vi "Main_flow_full_mqtt.vi"() -> ()   [LabVIEW 2022 SP3]
uses:
  D:/UOM/EE2044 - Electrical Measurements and Instrumentation/Project/Measurment Project/Quaxo_MQTT_LabVIEW-master/Controls/QoS.ctl
  D:/UOM/EE2044 - Electrical Measurements and Instrumentation/Project/Measurment Project/Quaxo_MQTT_LabVIEW-master/Controls/Retain_Flag.ctl
  D:/UOM/EE2044 - Electrical Measurements and Instrumentation/Project/Measurment Project/Quaxo_MQTT_LabVIEW-master/Controls/DUP_Flag.ctl
  D:/UOM/EE2044 - Electrical Measurements and Instrumentation/Project/Measurment Project/Quaxo_MQTT_LabVIEW-master/Controls/Connection_Return_Codes.ctl
  D:/UOM/EE2044 - Electrical Measurements and Instrumentation/Project/Measurment Project/Quaxo_MQTT_LabVIEW-master/Controls/Connect_Flags.ctl
  D:/UOM/EE2044 - Electrical Measurements and Instrumentation/Project/Measurment Project/Quaxo_MQTT_LabVIEW-master/Controls/User_Info.ctl
  <vilib>/DAQmx/write.llb/DAQmx Write (Digital Bool 1Line 1Point).vi
  <vilib>/DAQmx/read.llb/DAQmx Read (Digital Bool 1Line 1Point).vi
  <vilib>/DAQmx/read.llb/DAQmx Read (Analog 1D DBL NChan 1Samp).vi
  <vilib>/DAQmx/create/channels.llb/DAQmx Create Channel (AI-Voltage-Basic).vi
  <vilib>/DAQmx/create/channels.llb/DAQmx Create Channel (DO-Digital Output).vi
  <vilib>/DAQmx/create/channels.llb/DAQmx Create Channel (DI-Digital Input).vi
  <vilib>/DAQmx/miscellaneous.llb/DAQmx Fill In Error Info.vi
  D:/UOM/EE2044 - Electrical Measurements and Instrumentation/Project/Measurment Project/Quaxo_MQTT_LabVIEW-master/MQTT_Functions.lvlib
panel:
  out "Connection Status":T1=enum."Connection refused: not authorized"
  in  "Stop Publishing":bool
  out "Message published":string
  out "Acknowledged":bool
  out "Message ID (acknowledged)":u16=10
  in  "Message ID":u16=20
  in  "MQTT Broker":cluster{"address (IP)":string, "port":u16}={"address (IP)"="broker.mqttdashboard.com", "port"=1883}
  in  "Message to be published":string="Quaxo says it's "
  out "error out":errorcluster
  in  "Client ID":string="NodeE-12345"
  in  "error in (no error)":errorcluster
  in  "Topic":string="testtopic/Node12345"
  in  "Publish Meta":cluster{"QoS":T2, "Retain":T3, "DUP":T4}
  out "main loop executed":dbl
  out "Servo Angle":dbl(slide) scale=0.0..150.0
  in  "stop (F)":bool
  out "Square":dynamicdata(graph)
  in  "Frequency":dbl=50.0
  in  "Offset":dbl=2.5
  in  "Amplitude":dbl=2.5
  out "LDR Value":dbl
  in  "Relay 2":tag
  in  "Relay 1":tag
  out "Numeric 2":dbl
  out "Numeric":dbl
  in  "UP DOWN 2":tag
  in  "UP DOWN 1":tag
  in  "Buzzer":tag
  out "Counter":dbl
  out "OUT COUNT":dbl
  out "IN COUNT":dbl
  in  "Door IR 1 & 2 & LDR":tag
  in  "Trigger Period(sec)":dbl
  out "Current Time":dbl
  in  "Mode":dbl
  in  "stop":bool
  # "Dev1/ai4:6"
  # "Dev1/port0/line2"
  # "Dev1/port0/line0"
  # "Dev1/port0/line1"
  # "Dev1/port0/line3"
  # "Dev1/port0/line3"
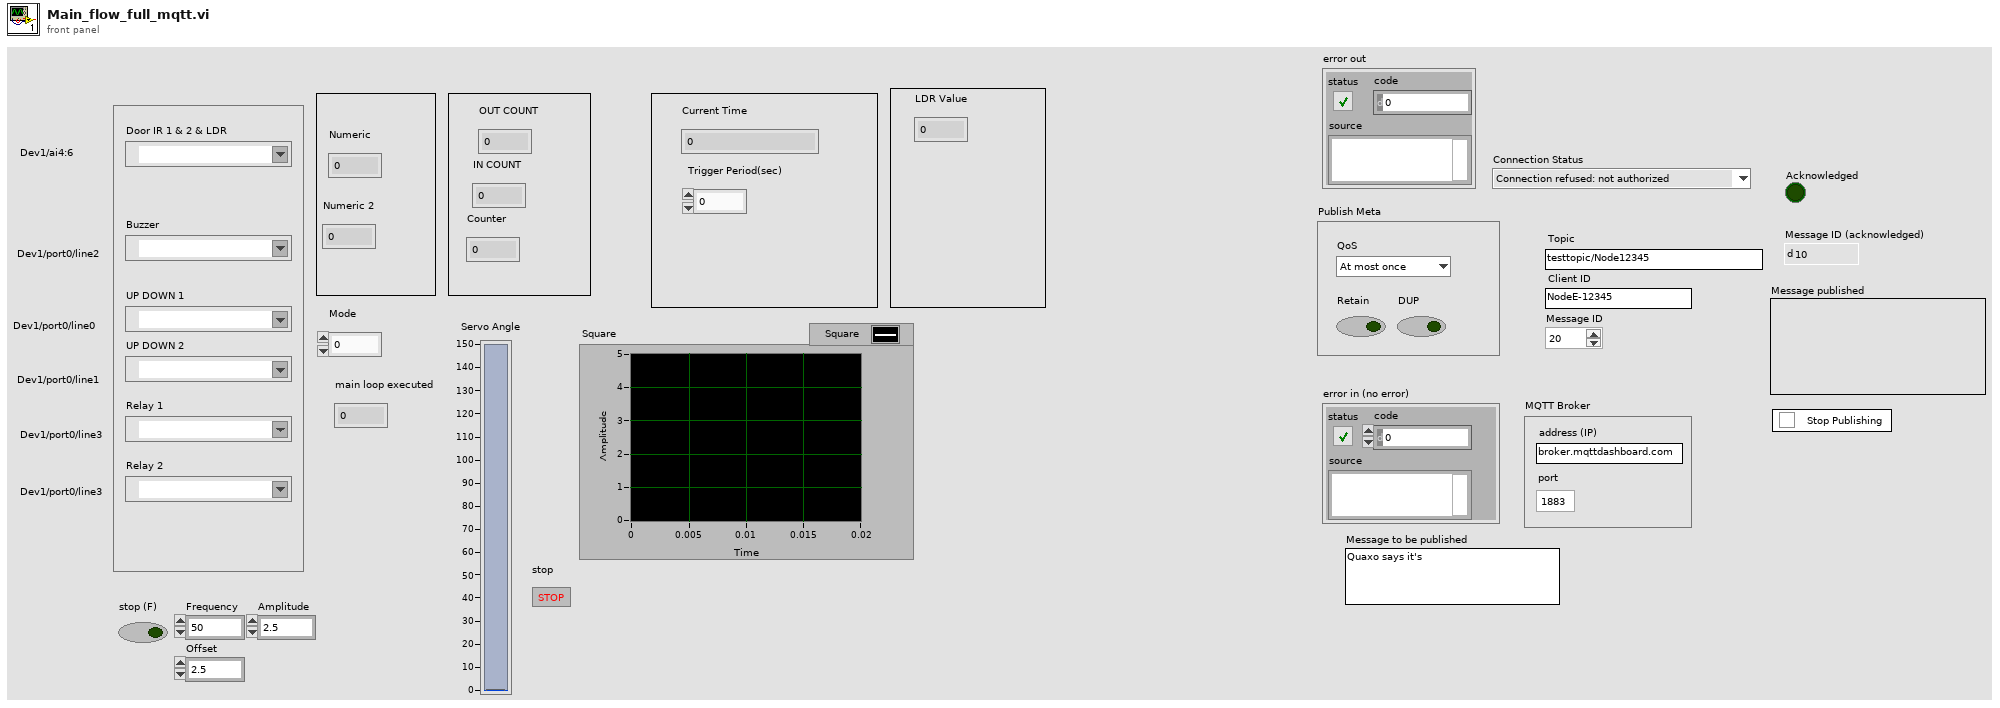
[diagram p1: front panel]
types:
  T1 = typedef "MQTT_Functions.lvlib/Connection_Return_Codes.ctl" = enum16{"Connection accepted", "Connection refused: unacceptable protocol version", "Connection refused: identifier rejected", "Connection refused: Server unavailable", "Connection refused: bad user name or password", "Connection refused: not authorized"}
  T2 = typedef "MQTT_Functions.lvlib/QoS.ctl" = enum8{"At most once", "At least once", "Exactly once", "Reserved"}
  T3 = typedef "MQTT_Functions.lvlib/Retain_Flag.ctl" = bool
  T4 = typedef "MQTT_Functions.lvlib/DUP_Flag.ctl" = bool
  T5 = typedef "MQTT_Functions.lvlib/User_Info.ctl" = cluster{"User Name":string, "Password":string}
  T6 = typedef "MQTT_Functions.lvlib/Connect_Flags.ctl" = cluster{"user name":bool, "password":bool, "will retain":bool, "will flag":bool, "clean session":bool, "reserved":bool, "will QoS":T2}
  T7 = cluster{"QoS":T2, "DUP":T4, "Retain":T3, "Keep Alive (sec)":u16}
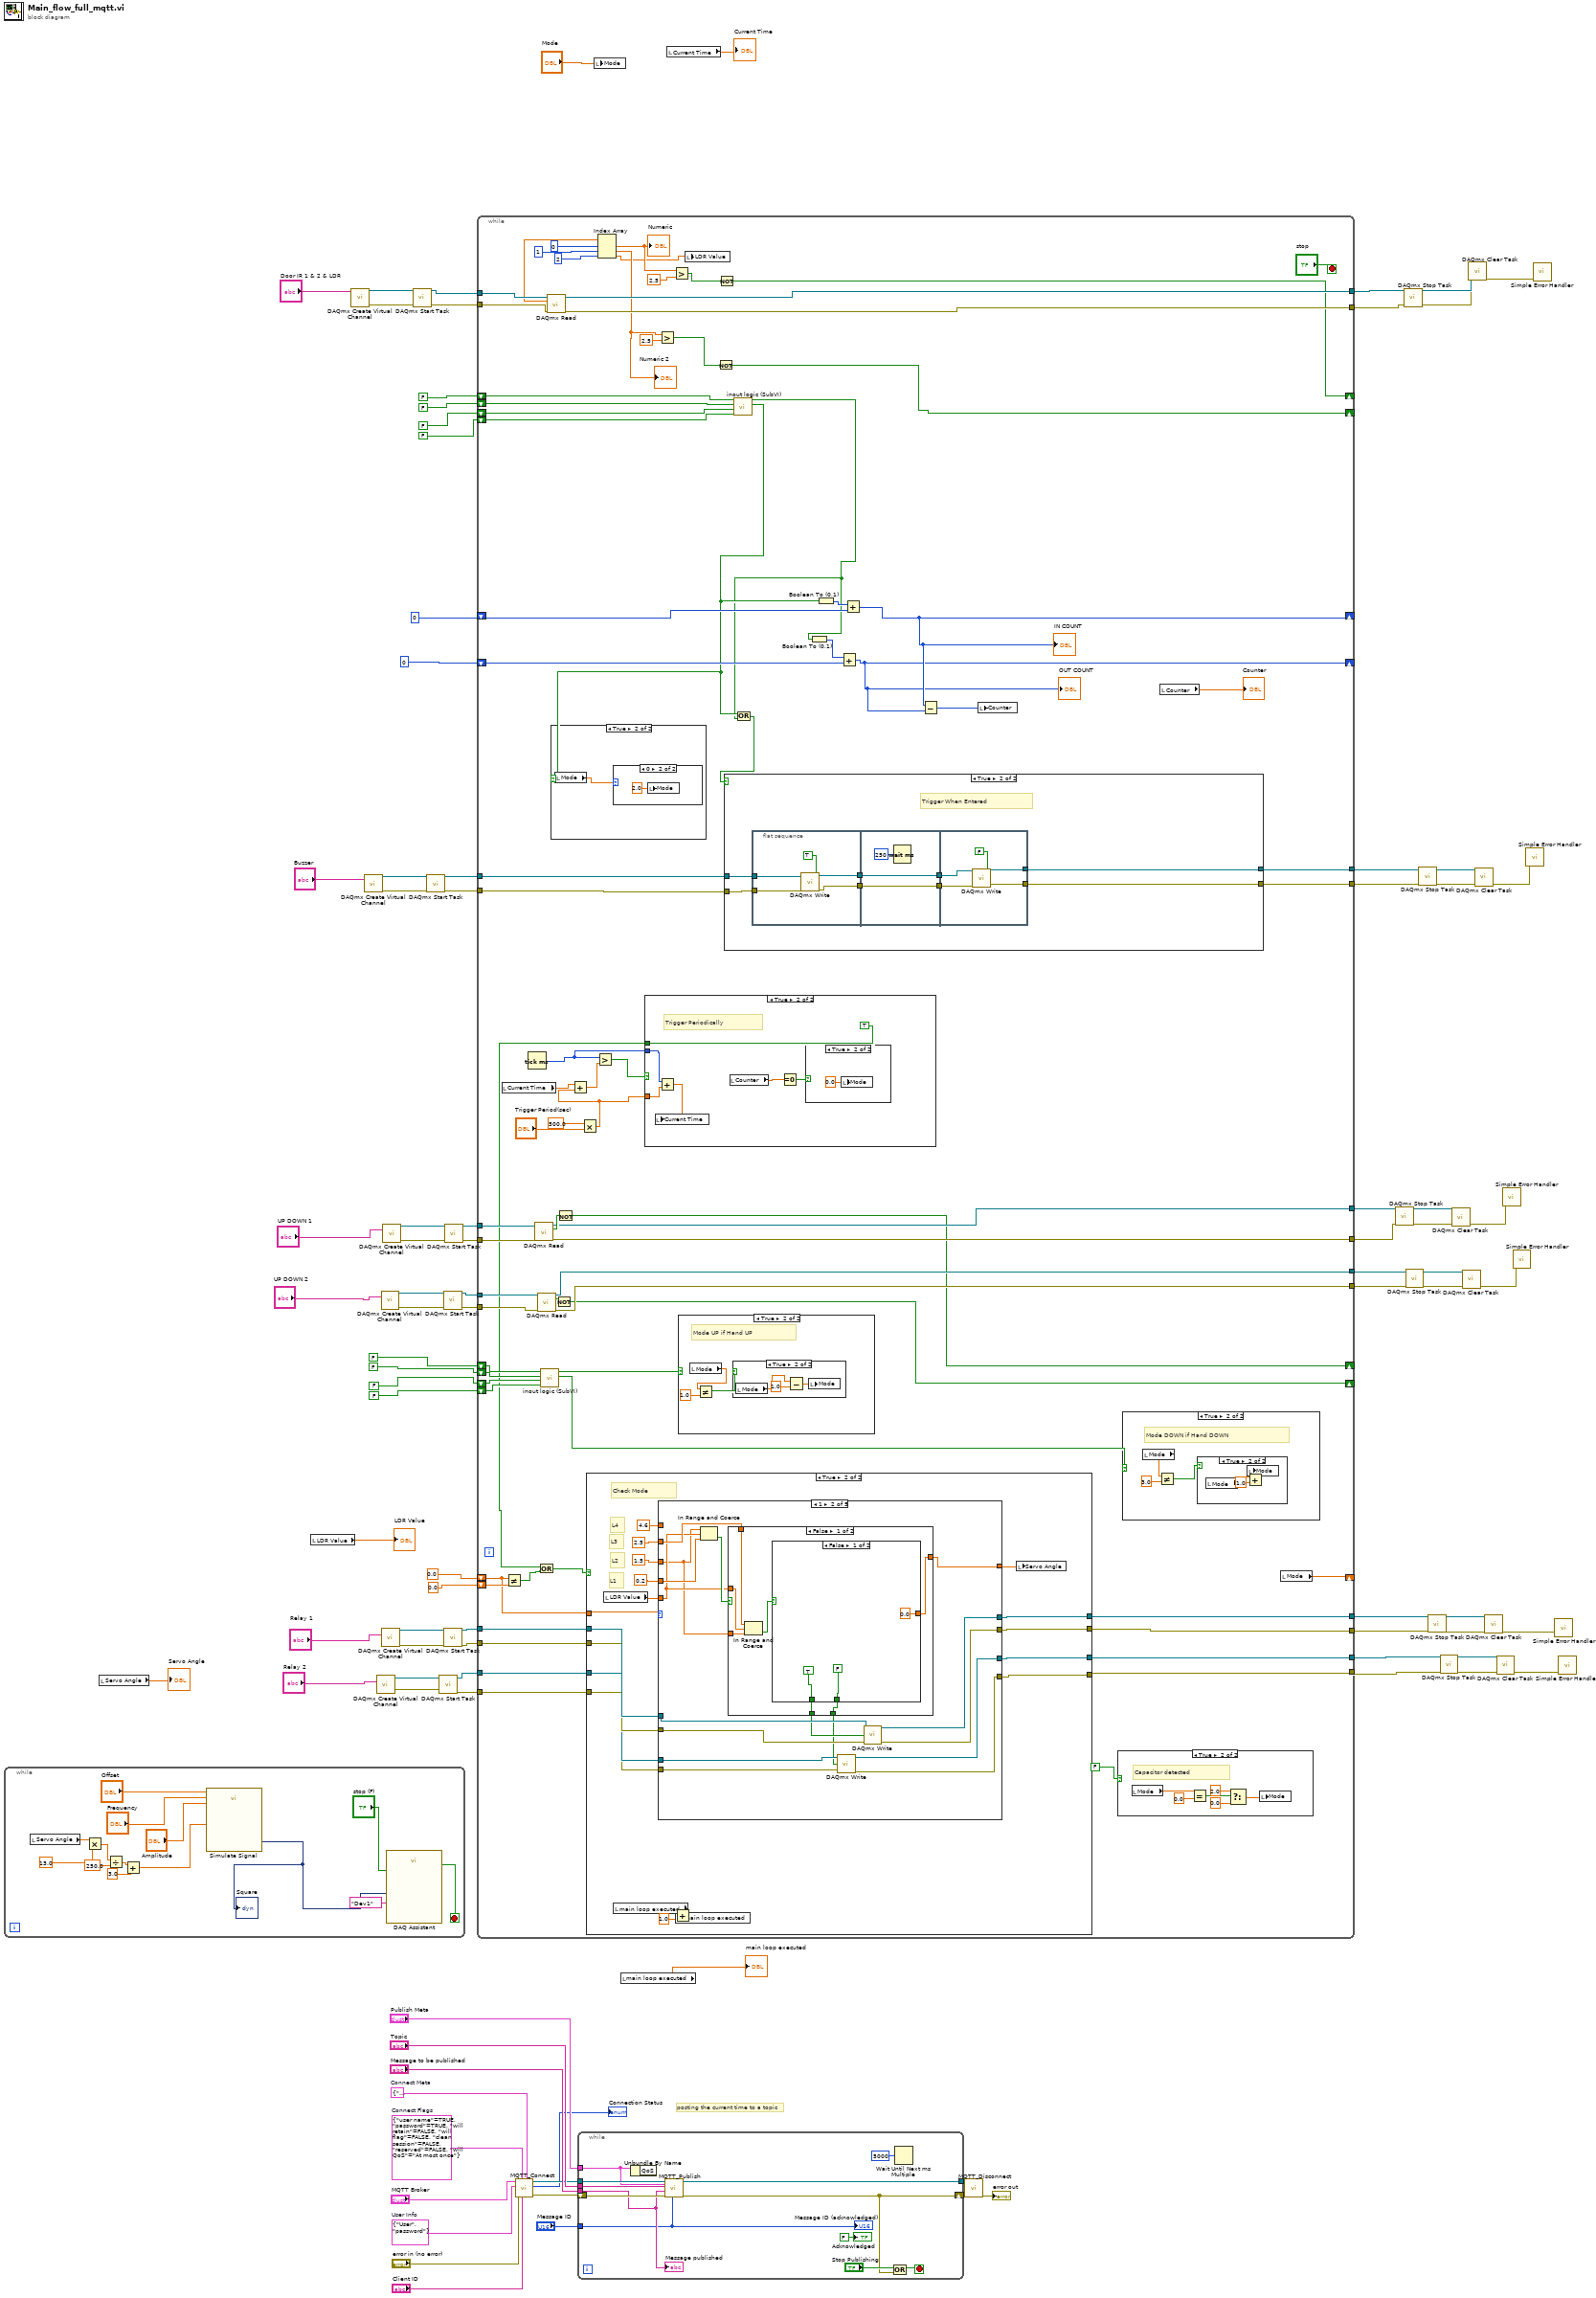
[diagram p0: block diagram]
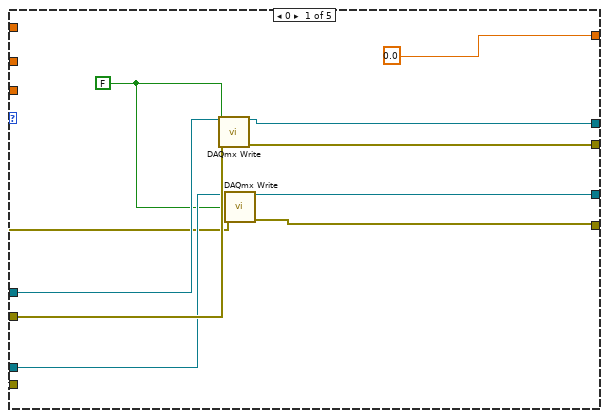
[diagram p5: hidden frame]
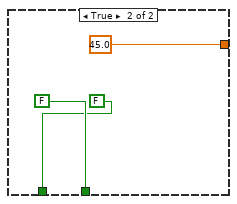
[diagram p6: hidden frame]
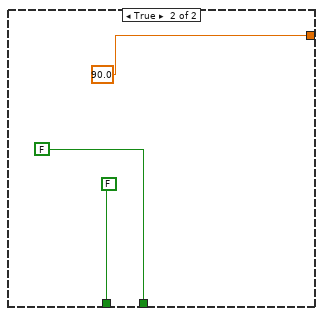
[diagram p7: hidden frame]
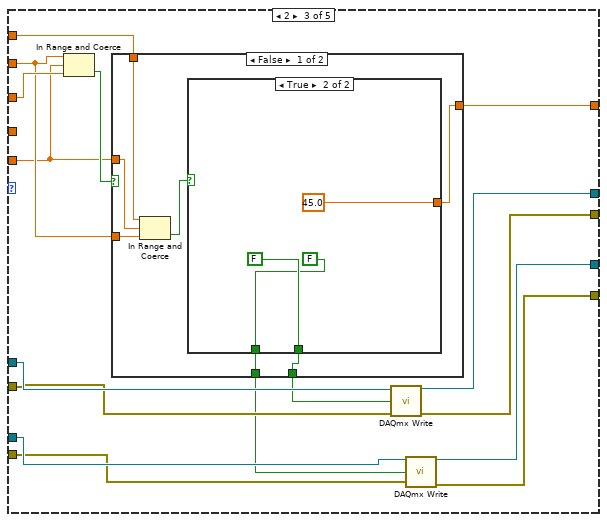
[diagram p8: hidden frame]
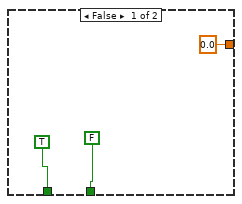
[diagram p9: hidden frame]
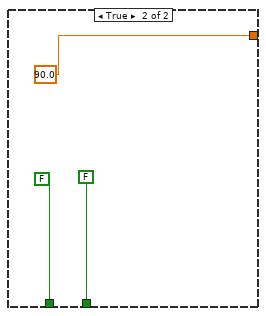
[diagram p10: hidden frame]
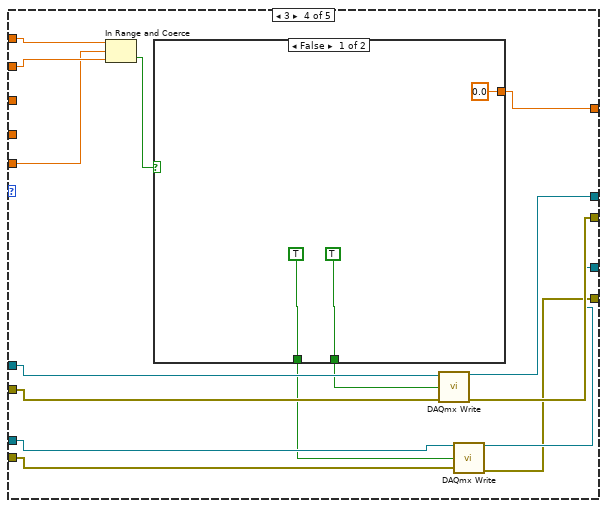
[diagram p11: hidden frame]
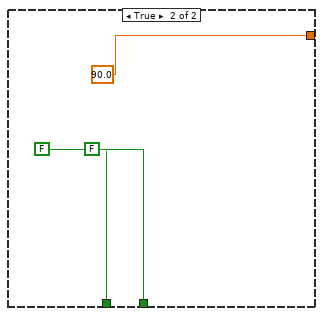
[diagram p12: hidden frame]
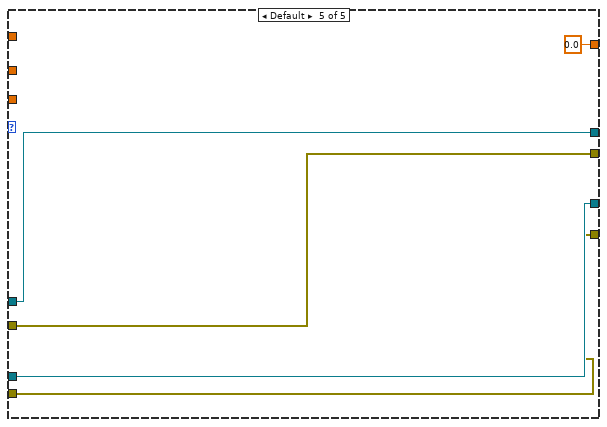
[diagram p13: hidden frame]
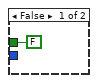
[diagram p18: hidden frame]
diagram:
  w2 = T5 {"User Name"="User", "Password"="password"}  # User Info
  w14 = T6 {"user name"=TRUE, "password"=TRUE, "will retain"=FALSE, "will flag"=FALSE, "clean session"=FALSE, "reserved"=FALSE, "will QoS"=enum."At most once"}  # Connect Flags
  w1 = T7 {"QoS"=enum."At most once", "DUP"=FALSE, "Retain"=FALSE, "Keep Alive (sec)"=60}  # Connect Meta
  # "posting the current time to a topic"
  n1 = while {
    stop <- w106 stop-if-true
    n2 = local read "Servo Angle"() -> (w94:dbl)
    n3 = Multiply(x=w94, y=13.0) -> (x*y=w100:dbl)
    n4 = Divide(x=w100, y=250.0) -> (x/y=w99:dbl)
    n5 = Add(x=w99, y=3.0) -> (x+y=w95:dbl)
    n6 = call "Simulate Signal"("Offset"="Offset", "Duty Cycle (%)"=w95, "Frequency"="Frequency", "Amplitude"="Amplitude") -> ("Square"=w102:dynamicdata)  [unwired: 10 in, 1 out]
    "Square" <- w102
    n7 = call "DAQ Assistant"("data"=w102, "stop (F)"="stop (F)", "device name"=tag "Dev1") -> ("stopped"=w106:bool)  [unwired: 14 in, 2 out]
  }
  n8 = local read "Servo Angle"() -> (→"Servo Angle":dbl)
  n9 = local read "LDR Value"() -> (→"LDR Value":dbl)
  n10 = call-poly <vilib>:"DAQmx Create Virtual Channel.vi"("physical channels"="Door IR 1 & 2 & LDR") -> ("task out"=w89:refnum<k21>, "error out"=w86:errorcluster)  [unwired: 13 in]
  n11 = call-poly <vilib>:"DAQmx Create Virtual Channel.vi"("lines"="Buzzer") -> ("task out"=w74:refnum<k21>, "error out"=w72:errorcluster)  [unwired: 13 in]
  n12 = call-poly <vilib>:"DAQmx Create Virtual Channel.vi"("lines"="Relay 2") -> ("task out"=w35:refnum<k21>, "error out"=w34:errorcluster)  [unwired: 13 in]
  n13 = call-poly <vilib>:"DAQmx Create Virtual Channel.vi"("lines"="UP DOWN 2") -> ("task out"=w63:refnum<k21>, "error out"=w61:errorcluster)  [unwired: 13 in]
  n14 = call-poly <vilib>:"DAQmx Create Virtual Channel.vi"("lines"="Relay 1") -> ("task out"=w38:refnum<k21>, "error out"=w37:errorcluster)  [unwired: 13 in]
  n15 = call-poly <vilib>:"DAQmx Create Virtual Channel.vi"("lines"="UP DOWN 1") -> ("task out"=w64:refnum<k21>, "error out"=w62:errorcluster)  [unwired: 13 in]
  n16 = call <vilib>:"DAQmx Start Task.vi"("task/channels in"=w89, "error in"=w86) -> ("task out"=w87:refnum<k21>, "error out"=w85:errorcluster)  [unwired: 12 in]
  n17 = call <vilib>:"DAQmx Start Task.vi"("task/channels in"=w74, "error in"=w72) -> ("task out"=w71:refnum<k21>, "error out"=w70:errorcluster)  [unwired: 12 in]
  n18 = call <vilib>:"DAQmx Start Task.vi"("task/channels in"=w35, "error in"=w34) -> ("task out"=w30:refnum<k21>, "error out"=w29:errorcluster)  [unwired: 12 in]
  n19 = call <vilib>:"DAQmx Start Task.vi"("task/channels in"=w63, "error in"=w61) -> ("task out"=w56:refnum<k21>, "error out"=w55:errorcluster)  [unwired: 12 in]
  n20 = call <vilib>:"DAQmx Start Task.vi"("task/channels in"=w38, "error in"=w37) -> ("task out"=w32:refnum<k21>, "error out"=w31:errorcluster)  [unwired: 12 in]
  n21 = call <vilib>:"DAQmx Start Task.vi"("task/channels in"=w64, "error in"=w62) -> ("task out"=w58:refnum<k21>, "error out"=w57:errorcluster)  [unwired: 12 in]
  n22 = while {
    shift-right: [w176] -> _
    shift-left: 0.0 ("Mode") -> [w174]
    shift-left: 0.0 ("Mode") -> [w175]
    tunnel: w87 -> [w171]
    tunnel: w85 -> [w170]
    tunnel: [w169] -> w84
    tunnel: [w168] -> w83
    shift-right: [w159] -> _
    shift-left: FALSE -> [w167]
    shift-left: FALSE -> [w166]
    shift-right: [w162] -> _
    shift-left: FALSE -> [w165]
    shift-left: FALSE -> [w136]
    shift-right: [w161] -> _
    shift-left: 0 -> [w164]
    shift-right: [w160] -> _
    shift-left: 0 -> [w163]
    tunnel: w71 -> [w156]
    tunnel: w70 -> [w155]
    tunnel: [w154] -> w66
    tunnel: [w153] -> w65
    shift-right: [w142] -> _
    shift-left: FALSE -> [w140]
    shift-right: [w141] -> _
    shift-left: FALSE -> [w138]
    shift-left: FALSE -> [w139]
    shift-left: FALSE -> [w137]
    tunnel: w58 -> [w150]
    tunnel: w57 -> [w149]
    tunnel: w56 -> [w148]
    tunnel: w55 -> [w147]
    tunnel: [w146] -> w48
    tunnel: [w145] -> w47
    tunnel: [w144] -> w46
    tunnel: [w143] -> w45
    tunnel: w32 -> [w118]
    tunnel: w31 -> [w117]
    tunnel: w30 -> [w116]
    tunnel: w29 -> [w115]
    tunnel: [w114] -> w22
    tunnel: [w113] -> w21
    tunnel: [w112] -> w20
    tunnel: [w111] -> w19
    stop <- "stop" stop-if-true
    n23 = local read "Current Time"() -> (w183:dbl)
    n24 = Not Equal?(x=w174, y=w175) -> (x != y?=w110:bool)
    n25 = Tick Count (ms)() -> (millisecond timer value=w181:u32)
    n26 = call-poly <vilib>:"DAQmx Read.vi"("task/channels in"=w150, "error in"=w149) -> ("task out"=w146:refnum<k21>, "data"=w152:bool, "error out"=w145:errorcluster)  [unwired: 11 in]
    n27 = call-poly <vilib>:"DAQmx Read.vi"("task/channels in"=w148, "error in"=w147) -> ("task out"=w144:refnum<k21>, "data"=w151:bool, "error out"=w143:errorcluster)  [unwired: 11 in]
    n28 = call "inout logic (SubVI).vi"("Sensor 2 (T-2)"=w137, "Sensor 2 (T-1)"=w138, "Sensor 1 (T-2)"=w139, "Sensor 1 (T-1)"=w140) -> ("IN"=w135:bool, "OUT"=w134:bool)  [unwired: 6 in]
    n29 = call-poly <vilib>:"DAQmx Read.vi"("task/channels in"=w171, "error in"=w170) -> ("task out"=w169:refnum<k21>, "data"=w128:dbl[], "error out"=w168:errorcluster)  [unwired: 11 in]
    n30 = Not(x=w151) -> (.not. x?=w141:bool)
    n31 = Not(x=w152) -> (.not. x?=w142:bool)
    n32 = Multiply(x=500.0, y="Trigger Period(sec)") -> (x*y=w177:dbl)
    n33 = Add(x=w183, y=w177) -> (x+y=w180:dbl)
    n34 = Greater?(x=w181, y=w180) -> (0:w182:bool)
    n35 = Index Array(array=w128, index #1=0 ("index"), index #2=1 ("index"), index #3=2 ("index")) -> (element #1=w127:dbl, element #2=w124:dbl, element #3=w119:dbl)
    "Numeric" <- w127
    "Numeric 2" <- w124
    n36 = case shown="True" w182 {
      tunnel: w181 -> [_ w326]
      tunnel: w177 -> [_ w325]
      tunnel: [FALSE ("Check") TRUE ("Check")] -> w108
      frame False {
      }
      frame True {
        # "Trigger Periodically"
        n37 = Add(x=w326, y=w325) -> (x+y=w327:dbl)
        n38 = local write "Current Time"(w327) -> ()
        n39 = local read "Counter"() -> (w324:dbl)
        n40 = Equal To 0?(x=w324) -> (x = 0?=w323:bool)
        n41 = case shown="True" w323 {
          frame False {
          }
          frame True {
            n42 = local write "Mode"(0.0 ("Mode")) -> ()
          }
        }
      }
    }
    n43 = Or(x=w108, y=w110) -> (x .or. y?=w109:bool)
    n44 = case shown="True" w109 {
      tunnel: w174 -> [_ w208]
      tunnel: w118 -> [w190 w207]
      tunnel: w117 -> [w189 w206]
      tunnel: w116 -> [w188 w205]
      tunnel: w115 -> [w187 w204]
      tunnel: [w190 w203] -> w114
      tunnel: [w189 w202] -> w113
      tunnel: [w188 w201] -> w112
      tunnel: [w187 w200] -> w111
      frame False {
      }
      frame True {
        # "L4"
        # "L1"
        # "L3"
        # "L2"
        # "Check Mode"
        n45 = local read "LDR Value"() -> (w198:dbl)
        n46 = local read "main loop executed"() -> (w193:dbl)
        n47 = case shown="1" w208 {
          tunnel: w207 -> [w218 w234 w266 w297 w308]
          tunnel: w206 -> [w217 w232 w265 w296 w307]
          tunnel: w205 -> [w216 w230 w264 w295 w306]
          tunnel: w204 -> [w215 w228 w263 w294 w305]
          tunnel: [w214 w233 w262 w293 w308] -> w203
          tunnel: [w213 w231 w261 w292 w307] -> w202
          tunnel: [w212 w229 w260 w291 w306] -> w201
          tunnel: [w211 w227 w259 w290 w305] -> w200
          tunnel: 1.5 -> [_ w222 w258 _ _]
          tunnel: 0.2 -> [_ w225 _ _ _]
          tunnel: w198 -> [_ w223 w251 w286 _]
          tunnel: 2.5 -> [_ w224 w252 w287 _]
          tunnel: 4.6 -> [_ _ w253 w288 _]
          tunnel: [0.0 ("Servo Angle") w219 w256 w285 0.0 ("A")] -> w194
          frame 0 {
            w210 = FALSE ("data")
            n48 = call-poly <vilib>:"DAQmx Write.vi"("task/channels in"=w218, "data"=w210, "error in"=w217) -> ("task out"=w214:refnum<k21>, "error out"=w213:errorcluster)  [unwired: 10 in, 1 out]
            n49 = call-poly <vilib>:"DAQmx Write.vi"("task/channels in"=w216, "data"=w210, "error in"=w215) -> ("task out"=w212:refnum<k21>, "error out"=w211:errorcluster)  [unwired: 10 in, 1 out]
          }
          frame 1 {
            n50 = In Range and Coerce(upper limit=w222, x=w223, lower limit=w225) -> (In Range?=w226:bool)  [unwired: 1 out]
            n51 = case shown="False" w226 {
              tunnel: [w237 90.0] -> w219
              tunnel: [w236 FALSE] -> w220
              tunnel: [w235 FALSE] -> w221
              tunnel: w224 -> [w241 _]
              tunnel: w222 -> [w240 _]
              tunnel: w223 -> [w239 _]
              frame False {
                n52 = In Range and Coerce(upper limit=w241, x=w239, lower limit=w240) -> (In Range?=w238:bool)  [unwired: 1 out]
                n53 = case shown="False" w238 {
                  tunnel: [0.0 45.0] -> w237
                  tunnel: [FALSE FALSE] -> w236
                  tunnel: [TRUE FALSE] -> w235
                  frame False {
                  }
                  frame True {
                  }
                }
              }
              frame True {
              }
            }
            n54 = call-poly <vilib>:"DAQmx Write.vi"("task/channels in"=w230, "data"=w220, "error in"=w228) -> ("task out"=w229:refnum<k21>, "error out"=w227:errorcluster)  [unwired: 10 in, 1 out]
            n55 = call-poly <vilib>:"DAQmx Write.vi"("task/channels in"=w234, "data"=w221, "error in"=w232) -> ("task out"=w233:refnum<k21>, "error out"=w231:errorcluster)  [unwired: 10 in, 1 out]
          }
          frame 2 {
            n56 = In Range and Coerce(upper limit=w252, x=w251, lower limit=w258) -> (In Range?=w257:bool)  [unwired: 1 out]
            n57 = case shown="False" w257 {
              tunnel: [w269 90.0] -> w256
              tunnel: [w268 FALSE] -> w255
              tunnel: [w267 FALSE] -> w254
              tunnel: w253 -> [w273 _]
              tunnel: w252 -> [w272 _]
              tunnel: w251 -> [w271 _]
              frame False {
                n58 = In Range and Coerce(upper limit=w273, x=w271, lower limit=w272) -> (In Range?=w270:bool)  [unwired: 1 out]
                n59 = case shown="True" w270 {
                  tunnel: [0.0 45.0] -> w269
                  tunnel: [FALSE FALSE] -> w268
                  tunnel: [TRUE FALSE] -> w267
                  frame False {
                  }
                  frame True {
                  }
                }
              }
              frame True {
              }
            }
            n60 = call-poly <vilib>:"DAQmx Write.vi"("task/channels in"=w266, "data"=w255, "error in"=w265) -> ("task out"=w262:refnum<k21>, "error out"=w261:errorcluster)  [unwired: 10 in, 1 out]
            n61 = call-poly <vilib>:"DAQmx Write.vi"("task/channels in"=w264, "data"=w254, "error in"=w263) -> ("task out"=w260:refnum<k21>, "error out"=w259:errorcluster)  [unwired: 10 in, 1 out]
          }
          frame 3 {
            n62 = In Range and Coerce(upper limit=w288, x=w286, lower limit=w287) -> (In Range?=w289:bool)  [unwired: 1 out]
            n63 = case shown="False" w289 {
              tunnel: [0.0 90.0] -> w285
              tunnel: [TRUE FALSE] -> w284
              tunnel: [TRUE FALSE] -> w283
              frame False {
              }
              frame True {
              }
            }
            n64 = call-poly <vilib>:"DAQmx Write.vi"("task/channels in"=w297, "data"=w284, "error in"=w296) -> ("task out"=w293:refnum<k21>, "error out"=w292:errorcluster)  [unwired: 10 in, 1 out]
            n65 = call-poly <vilib>:"DAQmx Write.vi"("task/channels in"=w295, "data"=w283, "error in"=w294) -> ("task out"=w291:refnum<k21>, "error out"=w290:errorcluster)  [unwired: 10 in, 1 out]
          }
          frame Default {
          }
        }
        n66 = Add(x=w193, y=1.0) -> (x+y=w191:dbl)
        n67 = local write "main loop executed"(w191) -> ()
        n68 = local write "Servo Angle"(w194) -> ()
      }
    }
    n69 = Greater?(x=w124, y=2.5) -> (0:w130:bool)
    n70 = Greater?(x=w127, y=2.5) -> (0:w132:bool)
    n71 = case shown="True" w134 {
      frame False {
      }
      frame True {
        # "Mode UP if Hand UP"
        n72 = local read "Mode"() -> (w311:dbl)
        n73 = Not Equal?(x=w311, y=1.0) -> (x != y?=w310:bool)
        n74 = case shown="True" w310 {
          frame False {
          }
          frame True {
            n75 = local read "Mode"() -> (w313:dbl)
            n76 = Subtract(x=w313, y=1.0) -> (x-y=w312:dbl)
            n77 = local write "Mode"(w312) -> ()
          }
        }
      }
    }
    n78 = local write "LDR Value"(w119) -> ()
    n79 = Not(x=w130) -> (.not. x?=w162:bool)
    n80 = Not(x=w132) -> (.not. x?=w159:bool)
    n81 = call "inout logic (SubVI).vi"("Sensor 2 (T-2)"=w136, "Sensor 2 (T-1)"=w165, "Sensor 1 (T-2)"=w166, "Sensor 1 (T-1)"=w167) -> ("IN"=w123:bool, "OUT"=w122:bool)  [unwired: 6 in]
    n82 = case shown="True" w123 {
      frame False {
      }
      frame True {
        n83 = local read "Mode"() -> (w185:dbl)
        n84 = case shown="0" w185 {
          frame Default {
          }
          frame 0 {
            n85 = local write "Mode"(2.0 ("Mode")) -> ()
          }
        }
      }
    }
    n86 = Or(x=w123, y=w122) -> (x .or. y?=w121:bool)
    n87 = case shown="True" w121 {
      tunnel: w156 -> [w329 w338]
      tunnel: w155 -> [w330 w337]
      tunnel: [w329 w332] -> w154
      tunnel: [w330 w331] -> w153
      frame False {
      }
      frame True {
        # "Trigger When Entered"
        n88 = flat-sequence {
          tunnel: w338 -> [w342]
          tunnel: w337 -> [w341]
          tunnel: [w340] -> w335
          tunnel: [w339] -> w333
          tunnel: [w345] -> w336
          tunnel: w335 -> [w345]
          tunnel: [w344] -> w334
          tunnel: w333 -> [w344]
          tunnel: w336 -> [w350]
          tunnel: w334 -> [w349]
          tunnel: [w348] -> w332
          tunnel: [w347] -> w331
          frame #0 {
            n89 = call-poly <vilib>:"DAQmx Write.vi"("task/channels in"=w342, "data"=TRUE, "error in"=w341) -> ("task out"=w340:refnum<k21>, "error out"=w339:errorcluster)  [unwired: 10 in, 1 out]
          }
          frame #1 {
            n90 = Wait (ms)(milliseconds to wait=u32 250) -> ()  [unwired: 1 out]
          }
          frame #2 {
            n91 = call-poly <vilib>:"DAQmx Write.vi"("task/channels in"=w350, "data"=FALSE, "error in"=w349) -> ("task out"=w348:refnum<k21>, "error out"=w347:errorcluster)  [unwired: 10 in, 1 out]
          }
        }
      }
    }
    n92 = Boolean To (0,1)(Boolean=w122) -> (0, 1=w172:i16)
    n93 = Boolean To (0,1)(Boolean=w123) -> (0, 1=w173:i16)
    n94 = Add(x=w172, y=w163) -> (x+y=w160:i32)
    "OUT COUNT" <- w160
    n95 = Add(x=w173, y=w164) -> (x+y=w161:i32)
    "IN COUNT" <- w161
    n96 = Subtract(x=w161, y=w160) -> (x-y=w158:i32)
    n97 = local write "Counter"(w158) -> ()
    n98 = case shown="True" FALSE {
      frame False {
      }
      frame True {
        # "Capacitor detected"
        n99 = local read "Mode"() -> (w357:dbl)
        n100 = Equal?(x=w357, y=0.0) -> (x = y?=w355:bool)
        n101 = Select(t=2.0, s=w355, f=0.0) -> (s? t:f=w354:dbl)
        n102 = local write "Mode"(w354) -> ()
      }
    }
    n103 = case shown="True" w135 {
      frame False {
      }
      frame True {
        # "Mode DOWN if Hand DOWN"
        n104 = local read "Mode"() -> (w317:dbl)
        n105 = Not Equal?(x=w317, y=3.0) -> (x != y?=w315:bool)
        n106 = case shown="True" w315 {
          frame False {
          }
          frame True {
            n107 = local read "Mode"() -> (w320:dbl)
            n108 = Add(x=w320, y=1.0) -> (x+y=w318:dbl)
            n109 = local write "Mode"(w318) -> ()
          }
        }
      }
    }
    n110 = local read "Counter"() -> (→"Counter":dbl)
    n111 = local read "Mode"() -> (w176:dbl)
  }
  n112 = call "MQTT_Connect.vi"("Connect Meta"=w1, "Client ID"="Client ID", "Connect Flags"=w14, "error in (no error)"="error in (no error)", "User Info"=w2, "MQTT Broker"="MQTT Broker") -> ("error out"=w3:errorcluster, "Connection Status"=→"Connection Status":T1, "connection ID out"=w5:refnum<k5>)  [unwired: 3 in]
  n113 = while {
    tunnel: "Topic" -> [w369]
    tunnel: "Message to be published" -> [w362]
    tunnel: w5 -> [w368]
    tunnel: "Publish Meta" -> [w366]
    tunnel: [w361] -> w8
    tunnel: "Message ID" -> [w358]
    shift-right: [w360] -> w9
    shift-left: w3 -> [w367]
    stop <- w364 stop-if-true
    n114 = Unbundle By Name(w366) -> ()  [unwired: 1 out]
    n115 = call "MQTT_Publish.vi"("Message ID"=w358, "Publish Meta"=w366, "error in (no error)"=w367, "Message to be published"=w362, "Topic"=w369, "connection ID"=w368) -> ("error out"=w360:errorcluster, "connection ID out"=w361:refnum<k5>)  [unwired: 4 in]
    n116 = Or(x="Stop Publishing", y=w360) -> (x .or. y?=w364:bool)
    n117 = Wait Until Next ms Multiple(millisecond multiple=u32 5000) -> ()  [unwired: 1 out]
    "Message published" <- w362
    "Acknowledged" <- FALSE ("Acknowledged")
    "Message ID (acknowledged)" <- w358
  }
  n118 = local write "Mode"("Mode") -> ()
  n119 = local read "main loop executed"() -> (→"main loop executed":dbl)
  n120 = local read "Current Time"() -> (→"Current Time":dbl)
  n121 = call "MQTT_Disconnect.vi"("error in (no error)"=w9, "connection ID"=w8) -> ("error out"=→"error out":errorcluster)  [unwired: 9 in]
  n122 = call <vilib>:"DAQmx Stop Task.vi"("task/channels in"=w48, "error in"=w47) -> ("task out"=w54:refnum<k21>, "error out"=w52:errorcluster)  [unwired: 12 in]
  n123 = call <vilib>:"DAQmx Stop Task.vi"("task/channels in"=w84, "error in"=w83) -> ("task out"=w82:refnum<k21>, "error out"=w81:errorcluster)  [unwired: 12 in]
  n124 = call <vilib>:"DAQmx Stop Task.vi"("task/channels in"=w46, "error in"=w45) -> ("task out"=w51:refnum<k21>, "error out"=w49:errorcluster)  [unwired: 12 in]
  n125 = call <vilib>:"DAQmx Stop Task.vi"("task/channels in"=w66, "error in"=w65) -> ("task out"=w69:refnum<k21>, "error out"=w67:errorcluster)  [unwired: 12 in]
  n126 = call <vilib>:"DAQmx Stop Task.vi"("task/channels in"=w22, "error in"=w21) -> ("task out"=w28:refnum<k21>, "error out"=w26:errorcluster)  [unwired: 12 in]
  n127 = call <vilib>:"DAQmx Stop Task.vi"("task/channels in"=w20, "error in"=w19) -> ("task out"=w25:refnum<k21>, "error out"=w23:errorcluster)  [unwired: 12 in]
  n128 = call <vilib>:"DAQmx Clear Task.vi"("task in"=w54, "error in"=w52) -> ("error out"=w53:errorcluster)  [unwired: 13 in]
  n129 = call <vilib>:"DAQmx Clear Task.vi"("task in"=w51, "error in"=w49) -> ("error out"=w50:errorcluster)  [unwired: 13 in]
  n130 = call <vilib>:"DAQmx Clear Task.vi"("task in"=w82, "error in"=w81) -> ("error out"=w80:errorcluster)  [unwired: 13 in]
  n131 = call <vilib>:"DAQmx Clear Task.vi"("task in"=w69, "error in"=w67) -> ("error out"=w68:errorcluster)  [unwired: 13 in]
  n132 = call <vilib>:"DAQmx Clear Task.vi"("task in"=w28, "error in"=w26) -> ("error out"=w27:errorcluster)  [unwired: 13 in]
  n133 = call <vilib>:"DAQmx Clear Task.vi"("task in"=w25, "error in"=w23) -> ("error out"=w24:errorcluster)  [unwired: 13 in]
  n134 = call <vilib>:"Simple Error Handler.vi"("error in (no error)"=w53) -> ()  [unwired: 4 in, 5 out]
  n135 = call <vilib>:"Simple Error Handler.vi"("error in (no error)"=w50) -> ()  [unwired: 4 in, 5 out]
  n136 = call <vilib>:"Simple Error Handler.vi"("error in (no error)"=w68) -> ()  [unwired: 4 in, 5 out]
  n137 = call <vilib>:"Simple Error Handler.vi"("error in (no error)"=w80) -> ()  [unwired: 4 in, 5 out]
  n138 = call <vilib>:"Simple Error Handler.vi"("error in (no error)"=w27) -> ()  [unwired: 4 in, 5 out]
  n139 = call <vilib>:"Simple Error Handler.vi"("error in (no error)"=w24) -> ()  [unwired: 4 in, 5 out]
